vi "Label Caption Visible read.vi"(9 "Ctl Refnum in":refnum<vi>) -> (1 "Caption.Visible":bool, 2 "Label.Visible":bool, 3 "Ctl Refnum out":refnum<vi>)   [LabVIEW 2010, in "Control.lvclass"]
uses:
  Control.lvclass
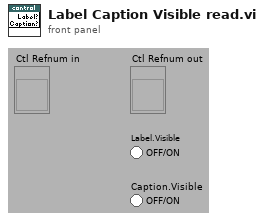
[diagram p1: front panel]
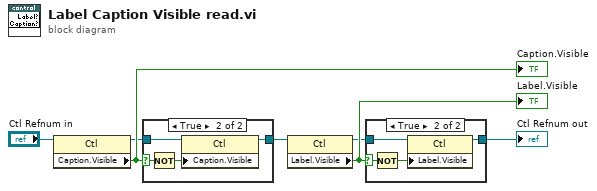
[diagram p0: block diagram]
diagram:
  n1 = property class="Ctl"(reference="Ctl Refnum in") -> (reference out=w2:refnum<vi>, "Caption.Visible"=w6:bool)  [unwired: 1 in, 1 out]
  "Caption.Visible" <- w6
  n2 = case shown="True" w6 {
    selector: w6 -> [_ w10]
    tunnel: w2 -> [w8 w12]
    tunnel: [w8 w11] -> w4
    frame False {
    }
    frame True {
      n3 = Not(x=w10) -> (.not. x?=w9:bool)
      n4 = property class="Ctl"(reference=w12, "Caption.Visible"=w9) -> (reference out=w11:refnum<vi>)  [unwired: 1 in, 1 out]
    }
  }
  n5 = property class="Ctl"(reference=w4) -> (reference out=w3:refnum<vi>, "Label.Visible"=w7:bool)  [unwired: 1 in, 1 out]
  "Label.Visible" <- w7
  n6 = case shown="True" w7 {
    selector: w7 -> [_ w15]
    tunnel: w3 -> [w13 w17]
    tunnel: [w13 w16] -> w5
    frame False {
    }
    frame True {
      n7 = Not(x=w15) -> (.not. x?=w14:bool)
      n8 = property class="Ctl"(reference=w17, "Label.Visible"=w14) -> (reference out=w16:refnum<vi>)  [unwired: 1 in, 1 out]
    }
  }
  "Ctl Refnum out" <- w5
